vi "Default Instrument Setup.vi"(8 "error in (no error)":errorcluster, 11 "VISA resource name":refnum<visa-resource-name>) -> (0 "error out":errorcluster, 3 "VISA resource name out":refnum<visa-resource-name>)   [LabVIEW 2026, in "Agilent 33XXX Series.lvlib"]
doc: "This Utility VI sends a default command string to the instrument whenever a new VISA session is opened, or the instrument is reset. Use this VI as a subVI for the <B>Initialize</B> and <B>Reset</B> VIs. Altering this VI could cause these two VIs to operate incorrectly."
uses:
  Agilent 33XXX Series.lvlib
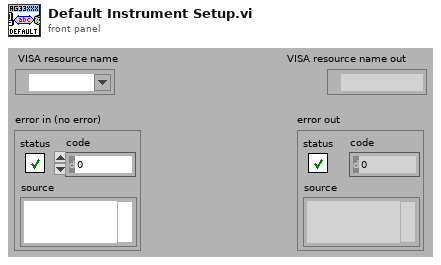
[diagram p1: front panel]
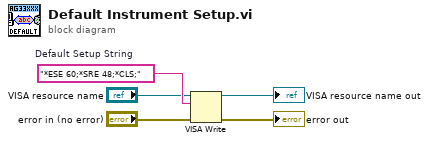
[diagram p0: block diagram]
diagram:
  w5 = "*ESE 60;*SRE 48;*CLS;"  # Default Setup String
  n1 = VISA Write(VISA resource name="VISA resource name", write buffer=w5, error in (no error)="error in (no error)") -> (VISA resource name out=→"VISA resource name out":refnum<visa-resource-name>, error out=→"error out":errorcluster)  [unwired: 1 out]
